vi "Is number even.vi"(11 "Number":i32) -> (1 "Even/Odd":enum16{"Number is even", "Number is odd"}(ring), 3 "Number (dup)":i32)   [LabVIEW 2017]
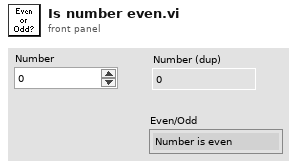
[diagram p1: front panel]
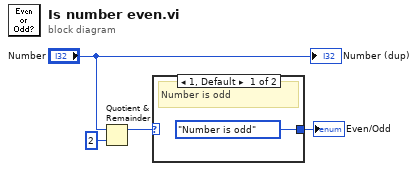
[diagram p0: block diagram]
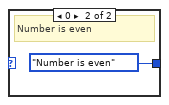
[diagram p2: hidden frame]
diagram:
  n1 = Quotient & Remainder(x="Number", y=2) -> (x-y*floor(x/y)=w4:i32)  [unwired: 1 out]
  n2 = case shown="1, Default" w4 {
    tunnel: [enum16{"Number is even", "Number is odd"}."Number is odd" ("Even/Odd") enum16{"Number is even", "Number is odd"}."Number is even" ("Even/Odd")] -> w2
    frame 1, Default {
      # "Number is odd"
    }
    frame 0 {
      # "Number is even"
    }
  }
  "Even/Odd" <- w2
  "Number (dup)" <- "Number"
